vi "samp_s3_2018.vi"() -> ()   [LabVIEW 2017]
uses:
  <userlib>/Open_device_2017.llb/Select_Instr.ctl
panel:
  out "error out":errorcluster
  out "Read counter":i32
  out "Opened":bool
  in  "stop":bool
  out "read buffer":string
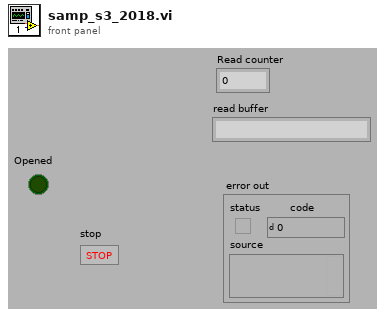
[diagram p1: front panel]
types:
  T1 = typedef "Select_Instr.ctl" = string
  T2 = cluster{"VISA resource name 1":refnum<visa-resource-name>, "VISA resource name 2":refnum<visa-resource-name>}
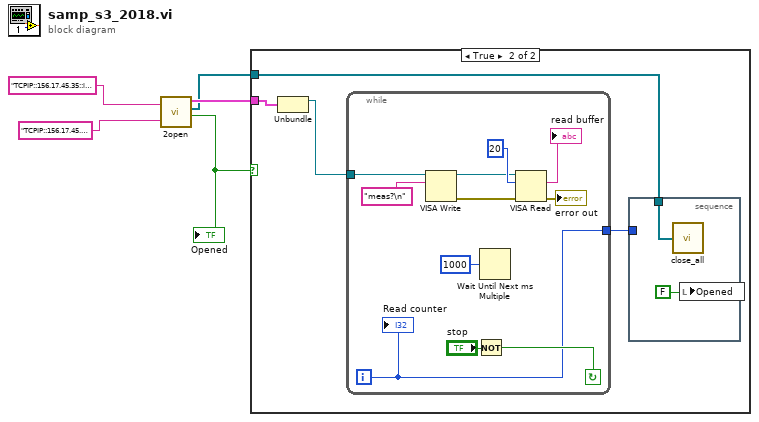
[diagram p0: block diagram]
diagram:
  n1 = call <userlib>:"2open.vi"("VISA resource name 1"=T1 "TCPIP::156.17.45.35::inst2::INSTR" ("Select_Instrument"), "VISA resource name 2"=T1 "TCPIP::156.17.45.35::inst1::INSTR" ("Select_Instrument")) -> ("InstrCluster"=w5:T2, "InstrArray"=w3:refnum<visa-resource-name>[], "Open OK (true)"=w4:bool)  [unwired: 1 out]
  "Opened" <- w4
  n2 = case shown="True" w4 {
    tunnel: w5 -> [_ w7]
    tunnel: w3 -> [_ w8]
    frame False {
    }
    frame True {
      n3 = Unbundle(w7) -> ("VISA resource name 1"=w6:refnum<visa-resource-name>)  [unwired: 1 out]
      n4 = while {
        tunnel: [w16] -> w9
        tunnel: w6 -> [w12]
        i -> [w16]
        stop <- w18 continue-if-true
        n5 = VISA Write(VISA resource name=w12, write buffer="meas?\n" ("write buffer (\"\")")) -> (VISA resource name out=w15:refnum<visa-resource-name>, error out=w14:errorcluster)  [unwired: 1 in, 1 out]
        n6 = Not(x="stop") -> (.not. x?=w18:bool)
        n7 = Wait Until Next ms Multiple(millisecond multiple=u32 1000) -> ()  [unwired: 1 out]
        n8 = VISA Read(VISA resource name=w15, byte count=u32 20 ("byte count (0)"), error in (no error)=w14) -> (read buffer=→"read buffer":string, error out=→"error out":errorcluster)  [unwired: 2 out]
        "Read counter" <- w16
      }
      n9 = stacked-sequence {
        tunnel: w9 -> [_]
        tunnel: w8 -> [w10]
        frame #0 {
          n10 = call "close_all.vi"("OpenRes"=w10) -> ()  [unwired: 1 out]
          n11 = local write "Opened"(FALSE) -> ()
        }
      }
    }
  }
